vi "MGI Find Closest Point.vi"(1 "Distance Metric (Standard)":T1, 2 "Y":dbl, 3 "X":dbl, 4 "XY Graph Data":cluster{"X":dbl[], "Y":dbl[]}) -> (0 "Index of Closest Point":i32)   [LabVIEW 2016]
doc: "Finds the index of the point in the input data that is closest to the given x and y coordinates. The optional input allows the user to use the city block metric (i.e. the sum of the distances in the x and y directions) instead of the standard distance measurement.\n\nAuthored by Thomas E. Henage\nsupport@mooregoodideas.com\nwww.mooregoodideas.com\n\nCopyright (c) 2010, Moore Good Ideas, Inc.\n\nAll rights reserved.\n\nRedistribution and use in source and binary forms, with or without modification, are permitted provided that the following conditions are met:\n\n * Redistributions of source code must retain the above copyright notice, this list of conditions and the following disclaimer.\n * Redistributions in binary form must reproduce the above copyright notice, this list of conditions and the following disclaimer in the documentation and/or other materials provided with the distribution.\n * Neither the name of Moore Good Ideas, Inc. nor the names of its contributors may be used to endorse or promote products derived from this software without specific prior written permission.\n\nTHIS SOFTWARE IS PROVIDED BY THE COPYRIGHT HOLDERS AND CONTRIBUTORS \"AS IS\" AND ANY EXPRESS OR IMPLIED WARRANTIES, INCLUDING, BUT NOT LIMITED TO, THE IMPLIED WARRANTIES OF MERCHANTABILITY AND FITNESS FOR A PARTICULAR PURPOSE ARE DISCLAIMED. IN NO EVENT SHALL THE COPYRIGHT OWNER OR CONTRIBUTORS BE LIABLE FOR ANY DIRECT, INDIRECT, INCIDENTAL, SPECIAL, EXEMPLARY, OR CONSEQUENTIAL DAMAGES (INCLUDING, BUT NOT LIMITED TO, PROCUREMENT OF SUBSTITUTE GOODS OR SERVICES; LOSS OF USE, DATA, OR PROFITS; OR BUSINESS INTERRUPTION) HOWEVER CAUSED AND ON ANY THEORY OF LIABILITY, WHETHER IN CONTRACT, STRICT LIABILITY, OR TORT (INCLUDING NEGLIGENCE OR OTHERWISE) ARISING IN ANY WAY OUT OF THE USE OF THIS SOFTWARE, EVEN IF ADVISED OF THE POSSIBILITY OF SUCH DAMAGE."
uses:
  <userlib>/_MGI/Coordinates/MGI Coordinate Proximity Enum.ctl
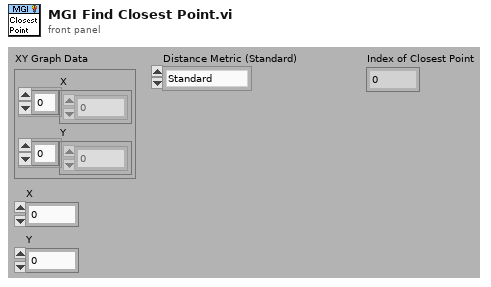
[diagram p1: front panel]
types:
  T1 = typedef "MGI Coordinate Proximity Enum.ctl" = enum16{"Standard", "City Block"}
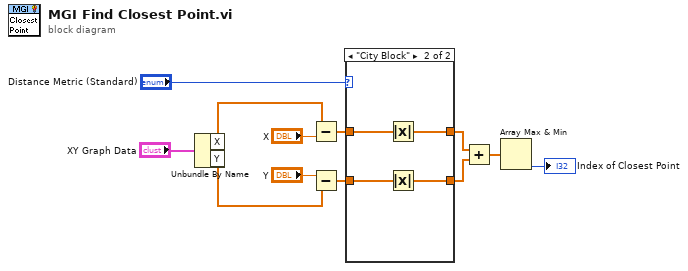
[diagram p0: block diagram]
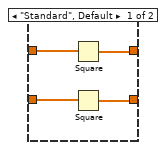
[diagram p2: hidden frame]
diagram:
  n1 = Unbundle By Name("XY Graph Data") -> ("X"=w4:dbl[], "Y"=w3:dbl[])
  n2 = Subtract(x=w4, y="X") -> (x-y=w7:dbl[])
  n3 = Subtract(x="Y", y=w3) -> (x-y=w8:dbl[])
  n4 = case shown="\"City Block\"" "Distance Metric (Standard)" {
    tunnel: [w16 w17] -> w10
    tunnel: [w15 w18] -> w9
    tunnel: w8 -> [w14 w19]
    tunnel: w7 -> [w13 w20]
    frame "Standard", Default {
      n5 = Square(x=w13) -> (x^2=w15:dbl[])
      n6 = Square(x=w14) -> (x^2=w16:dbl[])
    }
    frame "City Block" {
      n7 = Absolute Value(x=w20) -> (abs(x)=w18:dbl[])
      n8 = Absolute Value(x=w19) -> (abs(x)=w17:dbl[])
    }
  }
  n9 = Add(x=w9, y=w10) -> (x+y=w11:dbl[])
  n10 = Array Max & Min(array=w11) -> (min index (indices)=→"Index of Closest Point":i32)  [unwired: 3 out]
